vi "Read HART resource name.vi"(8 "error in (no error)":errorcluster, 11 "HART in":refnum<class "HART.lvclass">) -> (0 "error out":errorcluster, 2 "HART resource name":refnum<visa-resource-name>="HART", 3 "HART out":refnum<class "HART.lvclass">)   [LabVIEW 2016, in "HART.lvclass"]
uses:
  HART.lvclass
  HART.lvclass/HART.ctl
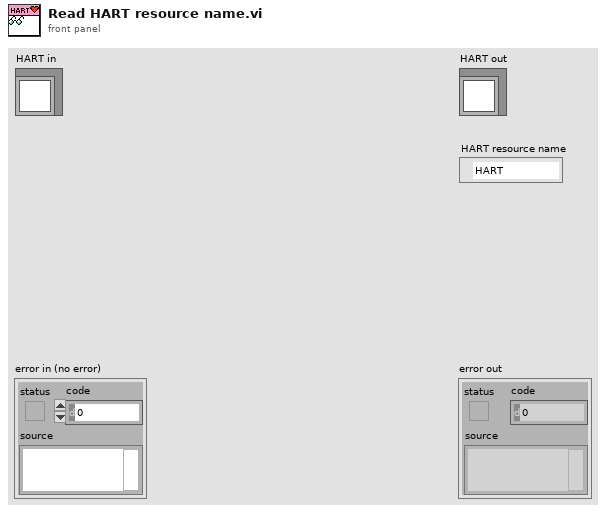
[diagram p1: front panel]
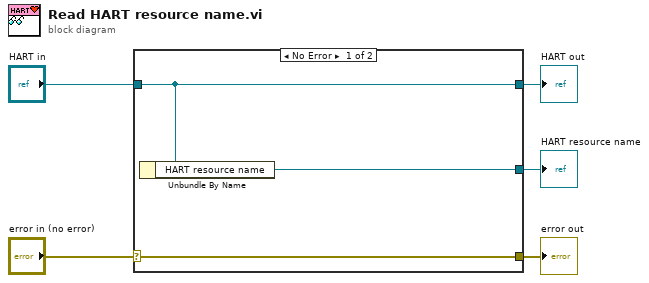
[diagram p0: block diagram]
diagram:
  n1 = case shown="No Error" "error in (no error)" {
    selector: "error in (no error)" -> [w8 w9]
    tunnel: [w8 w9] -> w4
    tunnel: [w7 w10] -> w2
    tunnel: "HART in" -> [w7 w10]
    tunnel: [w6 _] -> w1
    frame No Error {
      n2 = Unbundle By Name(w7) -> ("HART resource name"=w6:refnum<visa-resource-name>)
    }
    frame Error {
    }
  }
  "error out" <- w4
  "HART out" <- w2
  "HART resource name" <- w1
